vi "Read sensor inverts from config.vi"(8 "error in":errorcluster, 11 "Settings":variant) -> (0 "error out":errorcluster, 2 "Drive Sensors":T1, 3 "Settings out":variant)   [LabVIEW 2019, in "DriveOld.lvlib" / "Drive.lvclass"]
doc: "This VI reads the sensors inverts from the variant configuration and returns a type def."
uses:
  Drive.lvclass
  Controls/Drive Sensor Data.ctl
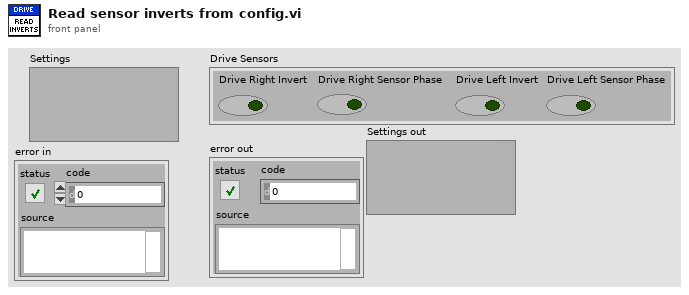
[diagram p1: front panel]
types:
  T1 = typedef "DriveOld.lvlib/Drive.lvclass/Drive Sensor Data.ctl" = cluster{"Drive Right Invert":bool, "Drive Right Sensor Phase":bool, "Drive Left Invert":bool, "Drive Left Sensor Phase":bool}
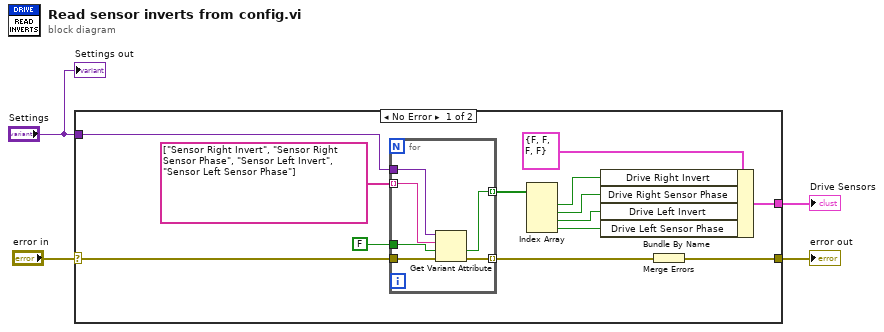
[diagram p0: block diagram]
diagram:
  n1 = case shown="No Error" "error in" {
    selector: "error in" -> [w5 w24]
    tunnel: [w17 w24] -> w4
    tunnel: "Settings" -> [w16 _]
    tunnel: [w7 _] -> w2
    frame No Error {
      n2 = for {
        tunnel: w16 -> [w23]
        tunnel: FALSE -> [w22]
        tunnel: [w21] -> w9 mode=indexing
        tunnel: [w20] -> w14 mode=indexing
        tunnel: string[] ["Sensor Right Invert", "Sensor Right Sensor Phase", "Sensor Left Invert", "Sensor Left Sensor Phase"] ("keys") -> [w19] mode=indexing
        tunnel: w5 -> [w18]
        n3 = Get Variant Attribute(Variant=w23, name=w19, default value (empty Variant)=w22, error in=w18) -> (value=w21:bool, error out=w20:errorcluster)  [unwired: 2 out]
      }
      n4 = Index Array(array=w9) -> (element #1=w10:bool, element #2=w11:bool, element #3=w12:bool, element #4=w13:bool)  [unwired: 4 in]
      n5 = Bundle By Name(cluster=T1 {"Drive Right Invert"=FALSE, "Drive Right Sensor Phase"=FALSE, "Drive Left Invert"=FALSE, "Drive Left Sensor Phase"=FALSE} ("Drive Sensors"), "Drive Right Invert"=w10, "Drive Right Sensor Phase"=w11, "Drive Left Invert"=w12, "Drive Left Sensor Phase"=w13) -> (w7:T1)
      n6 = Merge Errors(w14) -> (w17:errorcluster)
    }
    frame Error {
    }
  }
  "error out" <- w4
  "Drive Sensors" <- w2
  "Settings out" <- "Settings"
